vi "Initialize Open Weather Session.vi"(8 "Error In":errorcluster, 11 "Dashboard In":refnum<class "Dashboard.lvclass">) -> (0 "Error Out":errorcluster, 3 "Dashboard Out":refnum<class "Dashboard.lvclass">)   [LabVIEW 2019, in "Dashboard.lvclass"]
uses:
  Dashboard.lvclass
  <vilib>/Memosfet/OpenWeatherAPI/Open Weather Session/Public/Controls/Coordenates.ctl
  Accessors/Open Weather Session/Set Open Weather Session.vi
  Accessors/Processes/Get Processes.vi
  Display Manager/Accessors/Open Weather Session/Set Open Weather Session.vi
  Display Manager/Display Manager.lvclass
  Audio Analyzer/Audio Analyzer.lvclass
  Draw Frame/Draw Frame.lvclass
  Error Handling/Error Handling.lvclass
  Sequencer/Sequencer.lvclass
  <vilib>/Memosfet/OpenWeatherAPI/Open Weather Session/Open Weather Session.lvclass
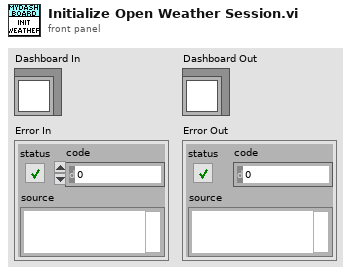
[diagram p1: front panel]
types:
  T1 = typedef "Open Weather Session.lvclass/Coordenates.ctl" = cluster{"Latitude":dbl, "Longitude":dbl}
  T2 = typedef "Dashboard.lvclass/Processes.ctl" = cluster{"Display Manager":refnum<class "Display Manager.lvclass">, "Audio Analyzer":refnum<class "Audio Analyzer.lvclass">, "Draw Frame":refnum<class "Draw Frame.lvclass">, "Error Handling":refnum<class "Error Handling.lvclass">, "Sequencer":refnum<class "Sequencer.lvclass">}
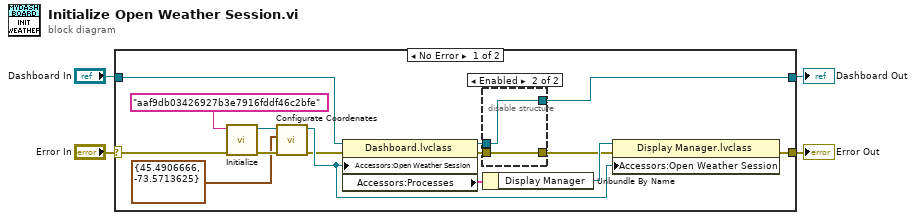
[diagram p0: block diagram]
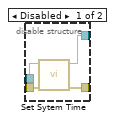
[diagram p2: hidden frame]
diagram:
  n1 = case shown="No Error" "Error In" {
    selector: "Error In" -> [w15 w27]
    tunnel: [w16 w27] -> w4
    tunnel: [w6 w26] -> w3
    tunnel: "Dashboard In" -> [w19 w26]
    frame No Error {
      n2 = call <vilib>:"Initialize.vi"("Error In"=w15, "API Key"="aaf9db03426927b3e7916fddf46c2bfe") -> ("Error Out"=w12:errorcluster, "Open Weather Session Out"=w13:refnum<class "Open Weather Session.lvclass">)  [unwired: 8 in]
      n3 = call-dynamic "Configurate Coordenates.vi"("Error In"=w12, "Coordenates"=T1 {"Latitude"=45.4906666, "Longitude"=-73.5713625}, "Open Weather Session In"=w13) -> ("Error Out"=w9:errorcluster, "Open Weather Session Out"=w10:refnum<class "Open Weather Session.lvclass">)  [unwired: 7 in]
      n4 = property class="Dashboard.lvclass"(reference=w19, error in=w9, "Accessors:Open Weather Session"=w10) -> (reference out=w7:refnum<class "Dashboard.lvclass">, error out=w8:errorcluster, "Accessors:Processes"=w18:T2)
      n5 = disable-structure shown="Enabled" {
        disable-tunnel: w8 -> [w23 w24]
        disable-tunnel: w7 -> [w22 w25]
        disable-tunnel: [w21 w25] -> w6
        disable-tunnel: [w20 w24] -> w5
        frame Disabled {
          n6 = call "Set Sytem Time.vi"("Error In"=w23, "Dashboard In"=w22) -> ("Error Out"=w20:errorcluster, "Dashboard Out"=w21:refnum<class "Dashboard.lvclass">)  [unwired: 8 in]
        }
        frame Enabled {
        }
      }
      n7 = Unbundle By Name(w18) -> ("Display Manager"=w17:refnum<class "Display Manager.lvclass">)
      n8 = property class="Display Manager.lvclass"(reference=w17, error in=w5, "Accessors:Open Weather Session"=w10) -> (error out=w16:errorcluster)  [unwired: 1 out]
    }
    frame Error {
    }
  }
  "Error Out" <- w4
  "Dashboard Out" <- w3
